vi "Vaisala Server.vi"(11 "DVR In":refnum<data-value>) -> (3 "DVR Out":refnum<data-value>)   [LabVIEW 2015]
uses:
  Data/Nicholas Data.lvclass
  Session/Raw FPGA/FPGA Session.lvclass
  Reusable/Session Log/System Log.lvclass
  Reusable/Session APIs/File Access/Config Data/Config Data.lvclass
  Session/FPGA Serial Session.lvclass
  Reusable/Data/Array Data/Single 1-D/Single_Array.lvclass
  Reusable/Session Log/System Log.lvclass/System Log.ctl
  Reusable/Session APIs/File Access/Config Data/Config Data.lvclass/Config Data.ctl
  Devices/Vaisala Probe/Vaisala.lvclass
  Devices/Vaisala Probe/Vaisala.lvclass/Vaisala.ctl
  Session/FPGA Serial Session.lvclass/FPGA Serial Session.ctl
  Reusable/Session APIs/Text Communication/Text Device Session.lvclass/Text Device Session.ctl
  Devices/Configurable Device/Configurable Device.lvclass/Configurable Device.ctl
  Data/Nicholas Data.lvclass/Nicholas Data.ctl
  Devices/Vaisala Probe/Accessors/Write ID.vi
  Session/Write fpgaSession.vi
  Reusable/Session APIs/Text Communication/Write hSysLog.vi
  Session/Write Timeout (ms).vi
  Devices/Configurable Device/Write Handle.vi
  Devices/Vaisala Probe/Accessors/Write hSession.vi
  Data/Write Vaisala Data.vi
  Reusable/Session APIs/File Access/Config Data/Accessors/Write Cfg Path.vi
  Reusable/Session Log/Accessors/Write Main Path.vi
  <userlib>/_Session Fwk/Session - Root.lvclass
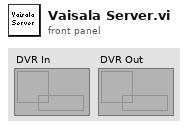
[diagram p1: front panel]
types:
  T1 = typedef "Session - Root.lvclass/Session Handle.ctl" = refnum<data-value>
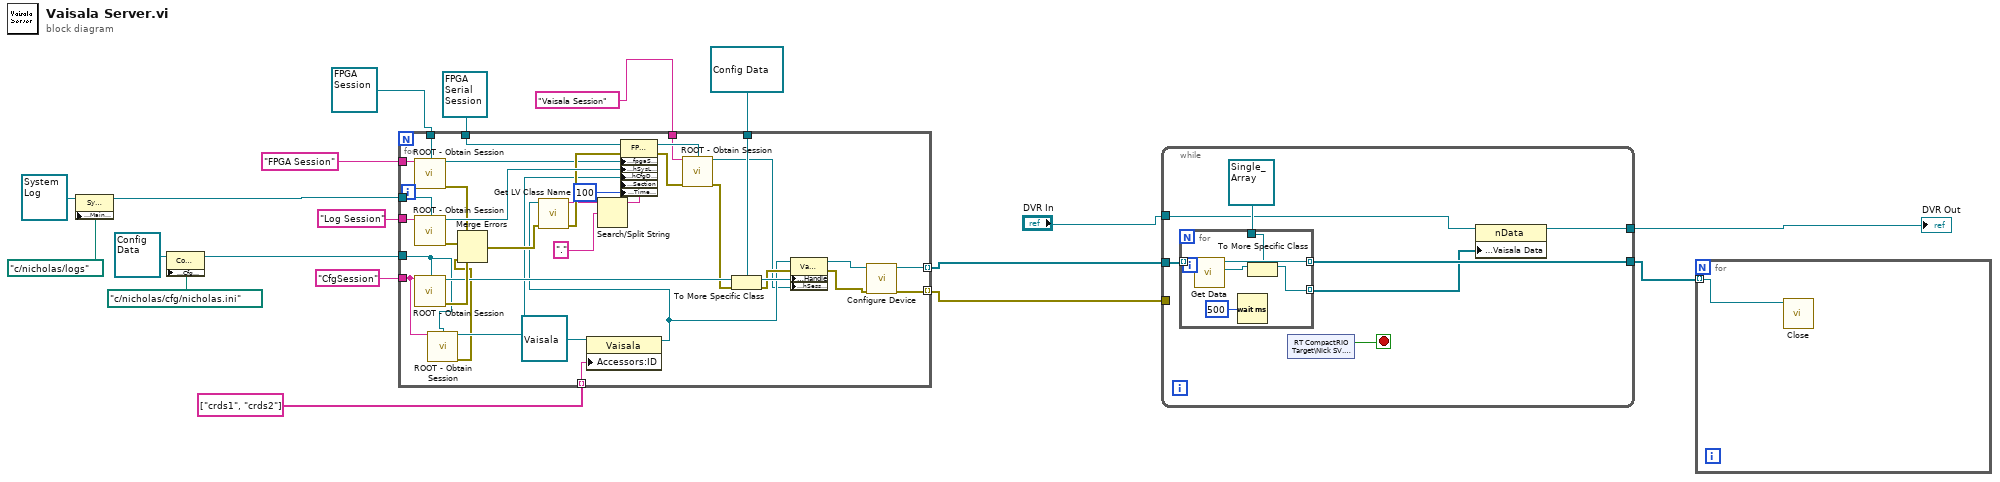
[diagram p0: block diagram]
diagram:
  n1 = property class="Sys Log"(reference=refnum<class "System Log.lvclass"> refnum ("Sys Log"), "Accessors:Main Path"=path "c:/nicholas/logs" ("Main Path")) -> (reference out=w9:refnum<class "System Log.lvclass">)  [unwired: 1 in, 1 out]
  n2 = property class="Config Data"(reference=refnum<class "Config Data.lvclass"> refnum ("Config Data"), "Accessors:Cfg Path"=path "c:/nicholas/cfg/nicholas.ini" ("Cfg Path")) -> (reference out=w10:refnum<class "Config Data.lvclass">)  [unwired: 1 in, 1 out]
  n3 = for {
    tunnel: w9 -> [w55]
    tunnel: "Log Session" ("Session Name ()") -> [w54]
    tunnel: refnum<class "FPGA Session.lvclass"> refnum ("FPGA Session") -> [w53]
    tunnel: "FPGA Session" ("Session Name ()") -> [w52]
    tunnel: w10 -> [w32]
    tunnel: "CfgSession" ("Session Name ()") -> [w33]
    tunnel: refnum<class "FPGA Serial Session.lvclass"> refnum ("FPGA Serial Session.lvclass") -> [w51]
    tunnel: refnum<data-value> refnum ("Session Handle") -> [w40]
    tunnel: "Vaisala Session" ("Session Name ()") -> [w34]
    tunnel: string[] ["crds1", "crds2"] -> [w26] mode=indexing
    tunnel: [w23] -> w7 mode=indexing
    tunnel: [w22] -> w3 mode=indexing
    n4 = call <userlib>:"ROOT - Obtain Session.vi"("Session Name ()"=w52, "OBJ - Session"=w53) -> ("Session Handle"=w20:T1, "error out"=w48:errorcluster)  [unwired: 11 in, 1 out]
    n5 = call <userlib>:"ROOT - Obtain Session.vi"("Session Name ()"=w54, "OBJ - Session"=w55) -> ("Session Handle"=w49:T1, "error out"=w47:errorcluster)  [unwired: 11 in, 1 out]
    n6 = call <userlib>:"ROOT - Obtain Session.vi"("Session Name ()"=w33, "OBJ - Session"=w32) -> ("Session Handle"=w44:T1, "error out"=w46:errorcluster)  [unwired: 11 in, 1 out]
    n7 = call <userlib>:"ROOT - Obtain Session.vi"("Session Name ()"=w33, "OBJ - Session"=w32) -> ("Session Handle"=w31:T1, "error out"=w30:errorcluster)  [unwired: 11 in, 1 out]
    n8 = Merge Errors(w48, w47, w46, w30) -> (w39:errorcluster)
    n9 = property class="Vaisala"(reference=refnum<class "Vaisala.lvclass"> refnum ("Vaisala"), "Accessors:ID"=w26) -> (reference out=w28:refnum<class "Vaisala.lvclass">)  [unwired: 1 in, 1 out]
    n10 = call <vilib>:"Get LV Class Name.vi"("error in (no error)"=w39, "object"=w28) -> ("error out"=w38:errorcluster, "class name"=w36:string)  [unwired: 8 in]
    n11 = Search/Split String(string=w36, search string/char (-)="." ("regular expression")) -> (substring before match=w35:string)  [unwired: 1 in, 2 out]
    n12 = property class="FPGA Serial Session"(reference=w51, error in=w38, "Accessors:fpgaSession"=w20, "Accessors:hSysLog"=w49, "Accessors:hCfgData"=w31, "Accessors:Section"=w35, "Accessors:Timeout (ms)"=100 ("Timeout (ms)")) -> (reference out=w50:refnum<class "FPGA Serial Session.lvclass">, error out=w45:errorcluster)
    n13 = call <userlib>:"ROOT - Obtain Session.vi"("Session Name ()"=w34, "OBJ - Session"=w50, "error in (no error)"=w45) -> ("Session Handle"=w27:T1, "error out"=w42:errorcluster)  [unwired: 10 in, 1 out]
    n14 = To More Specific Class(target class=w40, reference=w44, error in=w42) -> (specific class reference=w43:refnum<data-value>, error out=w41:errorcluster)
    n15 = property class="Vaisala"(reference=w28, error in=w41, "Accessors:Handle"=w43, "Accessors:hSession"=w27) -> (reference out=w25:refnum<class "Vaisala.lvclass">, error out=w24:errorcluster)
    n16 = call-dynamic "Configure Device.vi"("error in"=w24, "Vaisala Probe in"=w25) -> ("error out"=w22:errorcluster, "Vaisala Probe out"=w23:refnum<class "Vaisala.lvclass">)  [unwired: 8 in]
  }
  n17 = while {
    tunnel: w7 -> [w62]
    tunnel: [w61] -> w2
    tunnel: "DVR In" -> [w58]
    tunnel: [w57] -> w5
    tunnel: w3 -> [_]
    stop <- w60 stop-if-true
    n18 = for {
      tunnel: w62 -> [w68] mode=indexing
      tunnel: [w67] -> w61 mode=indexing
      tunnel: refnum<class "Single_Array.lvclass"> refnum ("Base Data Lib:[SGL]") -> [w65]
      tunnel: [w64] -> w56 mode=indexing
      n19 = call-dynamic "Get Data.vi"("Cfg Dev in"=w68) -> ("Data"=w66:refnum<class "Data.lvclass">, "Cfg Dev out"=w67:refnum<class "Vaisala.lvclass">)  [unwired: 8 in, 1 out]
      n20 = Wait (ms)(milliseconds to wait=u32 500) -> ()  [unwired: 1 out]
      n21 = To More Specific Class(target class=w65, reference=w66) -> (specific class reference=w64:refnum<class "Single_Array.lvclass">)  [unwired: 1 in, 1 out]
    }
    n22 = shared-variable "RT CompactRIO Target\\Nick SV.lvlib\\Stop"() -> (w60:bool)  [unwired: 1 in, 1 out]
    n23 = property class="nData"(reference=w58, "Accessors:Vaisala Data"=w56) -> (reference out=w57:refnum<data-value>)  [unwired: 1 in, 1 out]
  }
  "DVR Out" <- w5
  n24 = for {
    tunnel: w2 -> [w69] mode=indexing
    n25 = call-dynamic "Close.vi"("Cfg Dev in"=w69) -> ()  [unwired: 9 in, 2 out]
  }
